vi "Command_Turret_MoveToPosition.vi"(7 "Startup":bool, 9 "Timeout":dbl=5000.0, 10 "Speed":dbl=1.0, 11 "Goal_Position":dbl) -> (2 "Turret_Speed":dbl=-1.0, 4 "Reint":bool, 6 "Completed":bool)   [LabVIEW 2019]
uses:
  Auto Utilities/Command_Execution_State.ctl
  Subsystems/Sensing/Sensor_Values.vi
panel:
  in  "Acceptable_Error":dbl
  in  "Kp":dbl=0.05
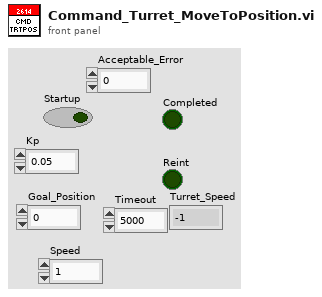
[diagram p1: front panel]
types:
  T1 = typedef "Command_Execution_State.ctl" = enum16{"Initialize", "Execute", "Finish"}
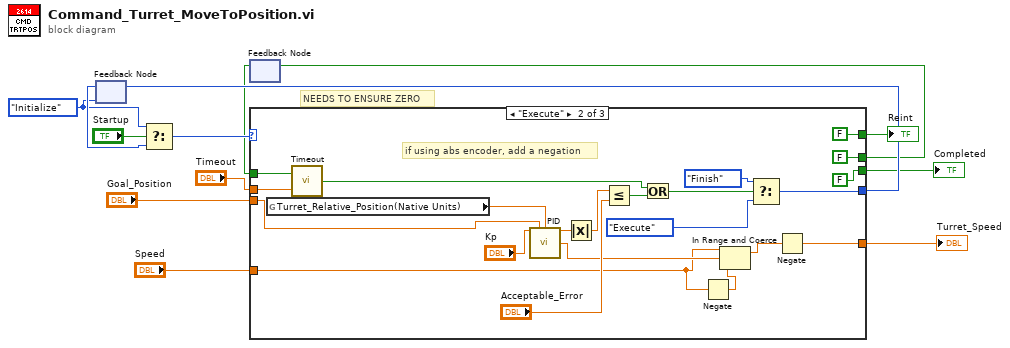
[diagram p0: block diagram]
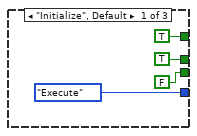
[diagram p2: hidden frame]
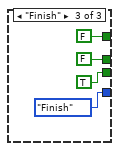
[diagram p3: hidden frame]
diagram:
  w7 = Command_Execution_State."Initialize" ("Play State")
  # "NEEDS TO ENSURE ZERO"
  n1 = feedback #1(w7) -> (w11:T1)
  n2 = Select(t=w7, s="Startup", f=w11) -> (s? t:f=w13:T1)
  n3 = feedback #2() -> (w4:bool)  [unwired: 1 in]
  n4 = case shown="\"Execute\"" w13 {
    tunnel: [Command_Execution_State."Execute" ("Play State") w32 Command_Execution_State."Finish" ("Play State")] -> w12
    tunnel: [FALSE FALSE TRUE] -> w10
    tunnel: [TRUE FALSE FALSE] -> w8
    tunnel: "Goal_Position" -> [_ w18 _]
    tunnel: w4 -> [_ w36 _]
    tunnel: [TRUE FALSE FALSE] -> w5
    tunnel: "Timeout" -> [_ w34 _]
    tunnel: [_ w20 _] -> w2
    tunnel: "Speed" -> [_ w22 _]
    frame "Initialize", Default {
    }
    frame "Execute" {
      # "if using abs encoder, add a negation"
      n5 = global read "Sensor_Values.vi" "Turret_Relative_Position(Native Units)"() -> (w19:dbl)
      n6 = call "Timeout.vi"("Timeout"=w34, "Initialize"=w36) -> ("Timed Out?"=w30:bool)
      n7 = call "PID.vi"("Kp"="Kp", "Process Variable"=w18, "Goal"=w19) -> ("Current Error"=w29:dbl, "Command"=w24:dbl)  [unwired: 10 in, 1 out]
      n8 = Absolute Value(x=w29) -> (abs(x)=w27:dbl)
      n9 = Less Or Equal?(x=w27, y="Acceptable_Error") -> (x <= y?=w28:bool)
      n10 = Or(x=w30, y=w28) -> (x .or. y?=w25:bool)
      n11 = Negate(x=w22) -> (-x=w23:dbl)
      n12 = In Range and Coerce(upper limit=w22, x=w24, lower limit=w23) -> (coerced(x)=w21:dbl)  [unwired: 1 out]
      n13 = Select(t=Command_Execution_State."Finish" ("Play State"), s=w25, f=Command_Execution_State."Execute" ("Play State")) -> (s? t:f=w32:T1)
      n14 = Negate(x=w21) -> (-x=w20:dbl)
    }
    frame "Finish" {
    }
  }
  "Completed" <- w10
  "Reint" <- w8
  "Turret_Speed" <- w2
  n15 = feedback-in #1(w12) -> ()
  n16 = feedback-in #2(w5) -> ()
